vi "Set RF Connection Direction.vi"(8 "error in (no error)":errorcluster, 9 "Direction (RX)":i32(ring) items=["RX", "TX", "TX & RX"], 10 "RF Connection (\"RF1.1\")":string="RF1.1", 11 "VISA resource name":refnum<visa-resource-name>) -> (0 "error out":errorcluster, 3 "VISA resource name out":refnum<visa-resource-name>)   [LabVIEW 2020, in "Rohde&Schwarz CMXP Base.lvlib"]
doc: "Defines the direction of a signal path (TX/RX of the instrument).\n\nAttribute:\n-\n\nRemote-control command:\n[CONFigure:]TENVironment:SPATh:DIRection"
uses:
  <instrlib>/Rohde&Schwarz CMXP Base/Rohde&Schwarz CMXP Base.lvlib
  <instrlib>/Rohde&Schwarz CMXP Base/Private/rsidr_core.llb/rsidr_core.lvlib
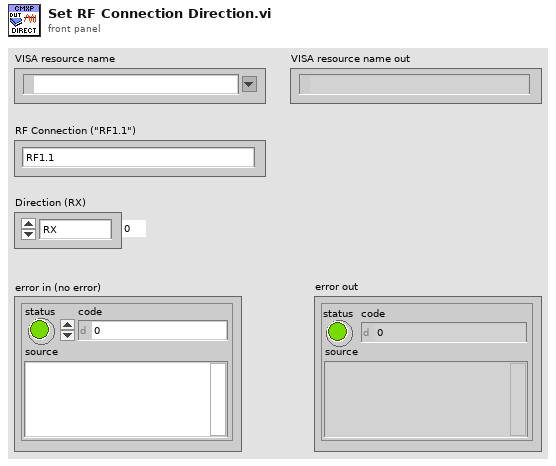
[diagram p1: front panel]
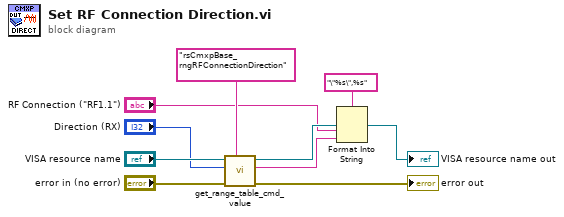
[diagram p0: block diagram]
diagram:
  n1 = call <instrlib>:"get_range_table_cmd_value.vi"("Range Table ID in"="rsCmxpBase_rngRFConnectionDirection", "error in"="error in (no error)", "Input Int32 value"="Direction (RX)", "VISA resource name"="VISA resource name") -> ("error out"=→"error out":errorcluster, "Cmd value out"=w1:string, "VISA resource name out"=→"VISA resource name out":refnum<visa-resource-name>)  [unwired: 5 in]
  n2 = Format Into String(format string="\"%s\",%s", "RF Connection (\"RF1.1\")", w1) -> ()  [unwired: 2 in, 2 out]
